vi "Query Measurements.vi"() -> ()   [LabVIEW 2024]
uses:
  <vilib>/Plug-In SDKs/Clients/Metadata/Outcome.ctl
  <vilib>/Plug-In SDKs/Clients/Data Store V1/Data Store Client.lvlibp
  <vilib>/Plug-In SDKs/Clients/Metadata/NI Metadata Types.lvlib
panel:
  out "All Measurements Count":i32
  out "Filtered Measurements":T2(array[cluster])
  out "All Measurements":T2(array[cluster])
  out "Filtered Measurements Count":i32
  in  "odata query":string="$filter=contains(Name,'Voltage')"
  out "error out":errorcluster
  # "Query Measurements"
  # "This example uses the Query Measurements API node with various odata filters to display different lists of measurements.\nRun Publish Data.vi to create the data and metadata queried by this VI."
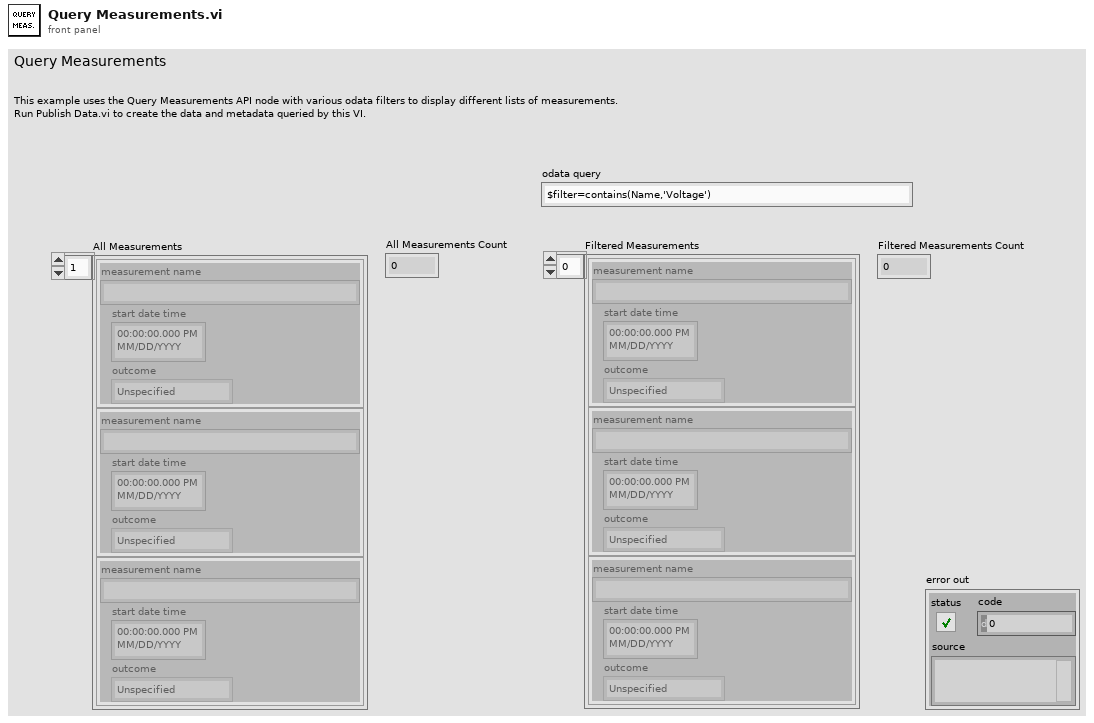
[diagram p1: front panel]
types:
  T1 = typedef "NI Metadata Types.lvlib/Outcome.ctl" = enum32{"Unspecified", "Passed", "Failed", "Indeterminate"}
  T2 = cluster{"measurement name":string, "start date time":timestamp, "outcome":T1}[]
  T3 = typedef "Data Store Client.lvlibp/Published Measurement.ctl" = cluster{"data moniker":T4, "published conditions":T5[], "published measurement id":string, "test result id":string, "step id":string, "software item ids":string[], "hardware item ids":string[], "test adapter ids":string[], "measurement name":string, "data type":string, "measurement notes":string, "start date time":timestamp, "end date time":timestamp, "outcome":T1, "parametric index":i32, "error information":T6}
  T4 = typedef "Data Store Client.lvlibp/Data Moniker.ctl" = cluster{"service location":string, "data source":string, "data instance":i64}
  T5 = typedef "Data Store Client.lvlibp/Published Condition.ctl" = cluster{"moniker":T4, "published condition id":string, "condition name":string, "condition type":string, "step id":string, "test result id":string}
  T6 = typedef "NI Metadata Types.lvlib/Error Information.ctl" = cluster{"error code":i32, "message":string, "source":string}
  T7 = cluster{"measurement name":string, "start date time":timestamp, "outcome":T1}
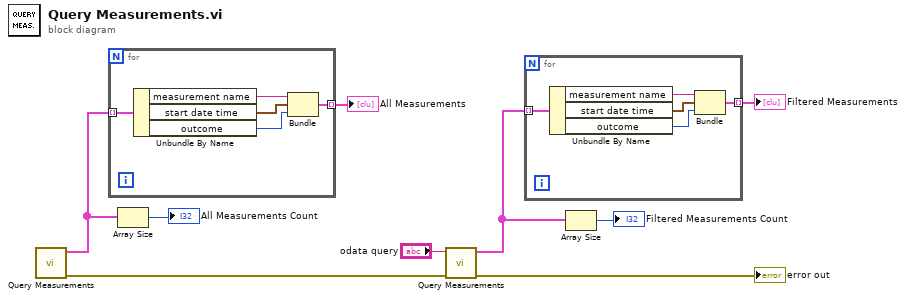
[diagram p0: block diagram]
diagram:
  n1 = call <vilib>:"Query Measurements.vi"() -> ("error out"=w4:errorcluster, "published measurements"=w1:T3[])  [unwired: 10 in]
  n2 = for {
    tunnel: w1 -> [w14] mode=indexing
    tunnel: [w11] -> w6 mode=indexing
    n3 = Unbundle By Name(w14) -> ("measurement name"=w13:string, "start date time"=w12:timestamp, "outcome"=w10:T1)
    n4 = Bundle("measurement name"=w13, "start date time"=w12, "outcome"=w10) -> (w11:T7)  [unwired: 1 in]
  }
  "All Measurements" <- w6
  n5 = Array Size(array=w1) -> (size(s)=→"All Measurements Count":i32)
  n6 = call <vilib>:"Query Measurements.vi"("error in"=w4, "odata query"="odata query") -> ("error out"=→"error out":errorcluster, "published measurements"=w8:T3[])  [unwired: 8 in]
  n7 = for {
    tunnel: w8 -> [w19] mode=indexing
    tunnel: [w16] -> w5 mode=indexing
    n8 = Unbundle By Name(w19) -> ("measurement name"=w18:string, "start date time"=w17:timestamp, "outcome"=w15:T1)
    n9 = Bundle("measurement name"=w18, "start date time"=w17, "outcome"=w15) -> (w16:T7)  [unwired: 1 in]
  }
  "Filtered Measurements" <- w5
  n10 = Array Size(array=w8) -> (size(s)=→"Filtered Measurements Count":i32)
